vi "SRV_PM_Trim Front of Unknown Packet Data_Simple.vi"(7 "1D Array":u8[](array[numeric])=[255, 255, 254, 255, 255, 255] format="%.0x", 9 "Search":u8[](array[numeric])=[255, 255, 255, 255] format="%.0x") -> (8 "Trimmed 1D Array":u8[](array[numeric]) format="%.0x")   [LabVIEW 2014]
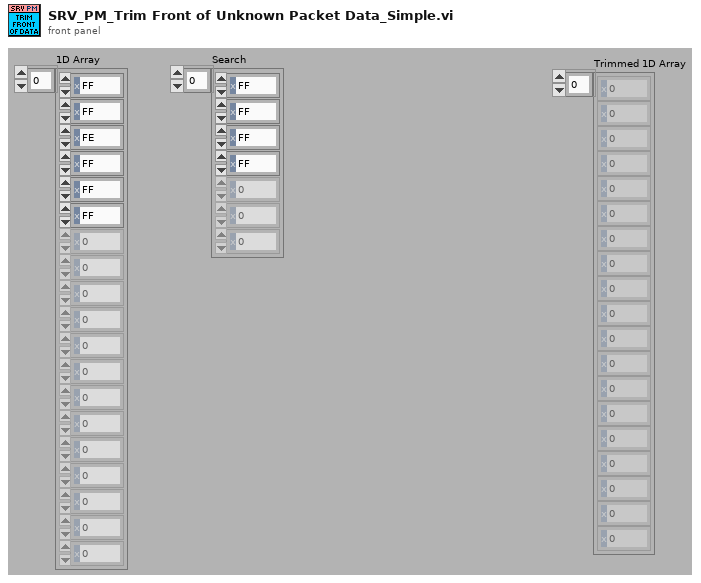
[diagram p1: front panel]
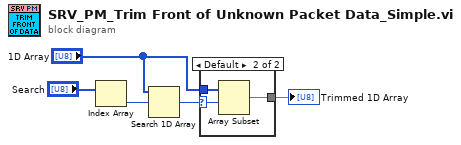
[diagram p0: block diagram]
diagram:
  n1 = Index Array(array="Search") -> (element=w5:u8)  [unwired: 1 in]
  n2 = Search 1D Array(1D array="1D Array", element=w5) -> (index of element=w3:i32)  [unwired: 1 in]
  n3 = case shown="Default" w3 {
    selector: w3 -> [_ w6]
    tunnel: "1D Array" -> [_ w8]
    tunnel: [_ w7] -> w1
    frame -1 {
    }
    frame Default {
      n4 = Array Subset(array=w8, index=w6) -> (w7:u8[])  [unwired: 1 in]
    }
  }
  "Trimmed 1D Array" <- w1
